vi "testTwoServersSendTelemetryAtSameTime.vi"(8 "error in":errorcluster) -> (0 "error out":errorcluster)   [LabVIEW 2018]
uses:
  <vilib>/addons/_JKI Toolkits/Caraya/classes/Assert/Assert Equal Value_Variant.vi
  src/TcpServer/TcpServer.lvclass
  <vilib>/addons/_JKI Toolkits/Caraya/classes/Test/Test.lvclass
  <vilib>/addons/_JKI Toolkits/Caraya/classes/Assert/Assert.lvclass
panel:
  out "Run Server B error":errorcluster
  out "Run Server A error":errorcluster
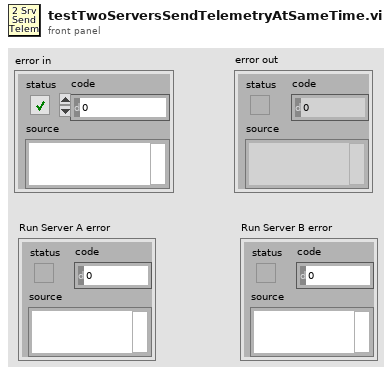
[diagram p1: front panel]
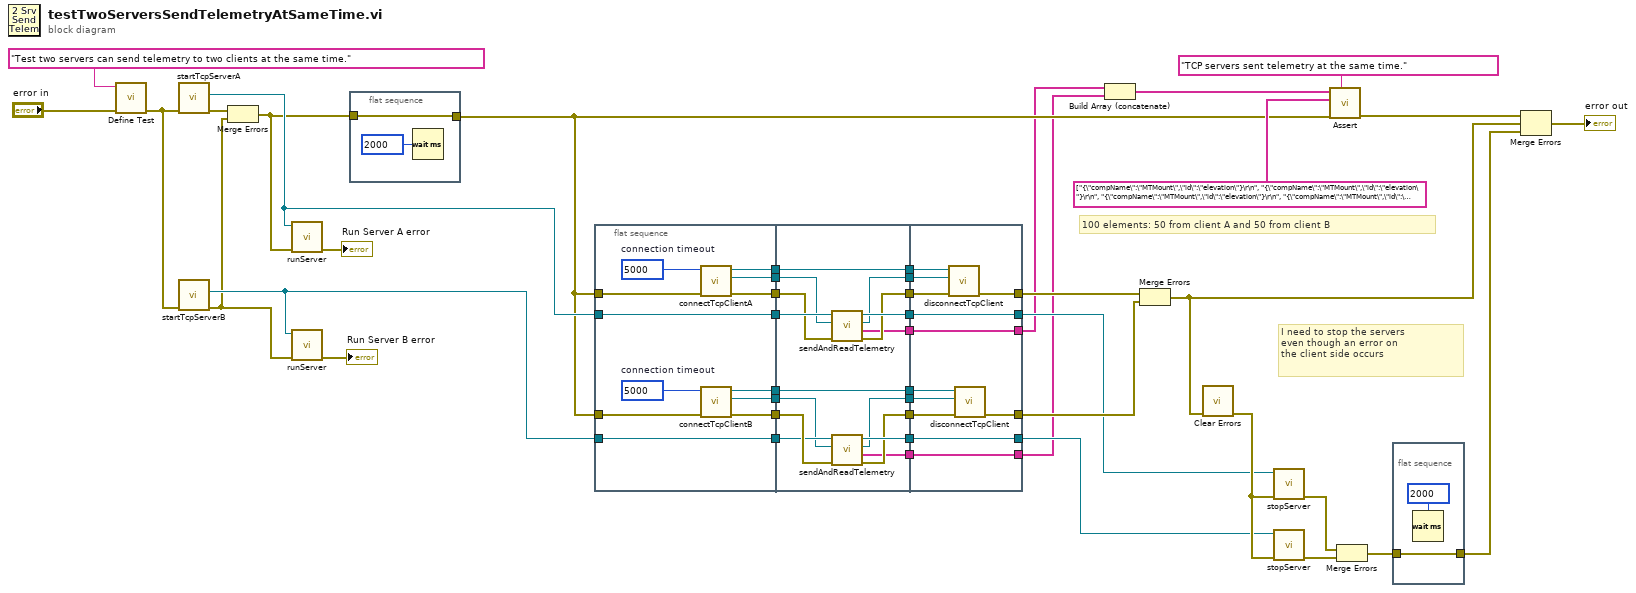
[diagram p0: block diagram]
diagram:
  # "100 elements: 50 from client A and 50 from client B"
  # "I need to stop the servers \neven though an error on \nthe client side occurs"
  n1 = call <vilib>:"Define Test.vi"("error in (no error)"="error in", "Label (VI Title)"="Test two servers can send telemetry to two clients at the same time.") -> ("error out"=w39:errorcluster)  [unwired: 9 in]
  n2 = call "startTcpServerA.vi"("error in (no error)"=w39) -> ("error out"=w35:errorcluster, "TcpServer out"=w34:refnum<class "TcpServer.lvclass">)  [unwired: 8 in, 1 out]
  n3 = call "startTcpServerB.vi"("error in (no error)"=w39) -> ("error out"=w1:errorcluster, "TcpServer out"=w33:refnum<class "TcpServer.lvclass">)  [unwired: 8 in, 1 out]
  n4 = Merge Errors(w35, w1) -> (w2:errorcluster)
  n5 = call "runServer.vi"("error in (no error)"=w2, "TcpServer in"=w34) -> ("error out (no error)"=→"Run Server A error":errorcluster)  [unwired: 8 in, 1 out]
  n6 = call "runServer.vi"("error in (no error)"=w1, "TcpServer in"=w33) -> ("error out (no error)"=→"Run Server B error":errorcluster)  [unwired: 8 in, 1 out]
  n7 = flat-sequence {
    tunnel: [w47] -> w24
    tunnel: w2 -> [w47]
    frame #0 {
      n8 = Wait (ms)(milliseconds to wait=u32 2000) -> ()  [unwired: 1 out]
    }
  }
  n9 = flat-sequence {
    tunnel: w33 -> [w59]
    tunnel: w34 -> [w60]
    tunnel: [w60] -> w29
    tunnel: [w59] -> w28
    tunnel: [w57] -> w27
    tunnel: w24 -> [w58]
    tunnel: [w56] -> w26
    tunnel: [w55] -> w25
    tunnel: w24 -> [w54]
    tunnel: [w53] -> w23
    tunnel: [w52] -> w22
    tunnel: [w51] -> w21
    tunnel: w29 -> [w74]
    tunnel: w28 -> [w69]
    tunnel: w27 -> [w72]
    tunnel: w26 -> [w73]
    tunnel: w25 -> [w76]
    tunnel: w23 -> [w70]
    tunnel: w22 -> [w75]
    tunnel: w21 -> [w67]
    tunnel: [w71] -> w18
    tunnel: [w68] -> w17
    tunnel: [w76] -> w16
    tunnel: [w75] -> w15
    tunnel: [w66] -> w14
    tunnel: [w65] -> w13
    tunnel: [w64] -> w12
    tunnel: [w63] -> w11
    tunnel: [w62] -> w10
    tunnel: [w61] -> w9
    tunnel: w18 -> [w80]
    tunnel: w17 -> [w78]
    tunnel: w16 -> [w86]
    tunnel: w15 -> [w83]
    tunnel: w14 -> [w84]
    tunnel: w13 -> [w81]
    tunnel: w12 -> [w85]
    tunnel: w11 -> [w82]
    tunnel: w10 -> [w79]
    tunnel: w9 -> [w77]
    tunnel: [w88] -> w8
    tunnel: [w87] -> w7
    tunnel: [w80] -> w6
    tunnel: [w79] -> w5
    tunnel: [w78] -> w4
    tunnel: [w77] -> w3
    frame #0 {
      w49 = 5000  # connection timeout
      w50 = 5000  # connection timeout
      n10 = call "connectTcpClientA.vi"("error in (no error)"=w58, "connection timeout (ms)"=w50) -> ("error out"=w57:errorcluster, "tel connection ID A out"=w56:refnum<k5>, "cmd connection ID A out"=w55:refnum<k5>)  [unwired: 7 in]
      n11 = call "connectTcpClientB.vi"("error in (no error)"=w54, "connection timeout (ms)"=w49) -> ("error out"=w53:errorcluster, "tel connection ID B out"=w51:refnum<k5>, "cmd connection ID B out"=w52:refnum<k5>)  [unwired: 7 in]
    }
    frame #1 {
      n12 = call "sendAndReadTelemetry.vi"("error in (no error)"=w72, "tel connection in"=w73, "TcpServer out"=w74) -> ("error out"=w66:errorcluster, "telemetry received"=w62:string[], "tel connection out"=w64:refnum<k5>, "tcpServer out"=w71:refnum<class "TcpServer.lvclass">)  [unwired: 5 in]
      n13 = call "sendAndReadTelemetry.vi"("error in (no error)"=w70, "tel connection in"=w67, "TcpServer out"=w69) -> ("error out"=w65:errorcluster, "telemetry received"=w61:string[], "tel connection out"=w63:refnum<k5>, "tcpServer out"=w68:refnum<class "TcpServer.lvclass">)  [unwired: 5 in]
    }
    frame #2 {
      n14 = call "disconnectTcpClient.vi"("error in (no error)"=w84, "tel connection ID in"=w85, "cmd connection ID in"=w86) -> ("error out"=w88:errorcluster)  [unwired: 8 in]
      n15 = call "disconnectTcpClient.vi"("error in (no error)"=w81, "tel connection ID in"=w82, "cmd connection ID in"=w83) -> ("error out"=w87:errorcluster)  [unwired: 8 in]
    }
  }
  n16 = Build Array (concatenate)(w5, w3) -> (w31:string[])
  n17 = Merge Errors(w8, w7) -> (w37:errorcluster)
  n18 = call <vilib>:"Clear Errors.vi"("error in (no error)"=w37) -> ("error out"=w36:errorcluster)  [unwired: 5 in, 1 out]
  n19 = call "stopServer.vi"("error in (no error)"=w36, "tcpServer in"=w6) -> ("error out"=w44:errorcluster)  [unwired: 8 in, 1 out]
  n20 = call "stopServer.vi"("error in (no error)"=w36, "tcpServer in"=w4) -> ("error out"=w43:errorcluster)  [unwired: 8 in, 1 out]
  n21 = call-poly <vilib>:"Assert.vi"("Label"="TCP servers sent telemetry at the same time.", "error in (no error)"=w24, "Y"=string[] ["{\"compName\":\"MTMount\",\"id\":\"elevation\"}\r\n", "{\"compName\":\"MTMount\",\"id\":\"elevation\"}\r\n", "{\"compName\":\"MTMount\",\"id\":\"elevation\"}\r\n", "{\"compName\":\"MTMount\",\"id\":\"elevation\"}\r\n", "{\"compName\":\"MTMount\",\"id\":\"elevation\"}\r\n", "{\"compName\":\"MTMount\",\"id\":\"elevation\"}\r\n", "{\"compName\":\"MTMount\",\"id\":\"elevation\"}\r\n", "{\"compName\":\"MTMount\",\"id\":\"elevation\"}\r\n", "{\"compName\":\"MTMount\",\"id\":\"elevation\"}\r\n", "{\"compName\":\"MTMount\",\"id\":\"elevation\"}\r\n", "{\"compName\":\"MTMount\",\"id\":\"elevation\"}\r\n", "{\"compName\":\"MTMount\",\"id\":\"elevation\"}\r\n", "{\"compName\":\"MTMount\",\"id\":\"elevation\"}\r\n", "{\"compName\":\"MTMount\",\"id\":\"elevation\"}\r\n", "{\"compName\":\"MTMount\",\"id\":\"elevation\"}\r\n", "{\"compName\":\"MTMount\",\"id\":\"elevation\"}\r\n", "{\"compName\":\"MTMount\",\"id\":\"elevation\"}\r\n", "{\"compName\":\"MTMount\",\"id\":\"elevation\"}\r\n", "{\"compName\":\"MTMount\",\"id\":\"elevation\"}\r\n", "{\"compName\":\"MTMount\",\"id\":\"elevation\"}\r\n", "{\"compName\":\"MTMount\",\"id\":\"elevation\"}\r\n", "{\"compName\":\"MTMount\",\"id\":\"elevation\"}\r\n", "{\"compName\":\"MTMount\",\"id\":\"elevation\"}\r\n", "{\"compName\":\"MTMount\",\"id\":\"elevation\"}\r\n", "{\"compName\":\"MTMount\",\"id\":\"elevation\"}\r\n", "{\"compName\":\"MTMount\",\"id\":\"elevation\"}\r\n", "{\"compName\":\"MTMount\",\"id\":\"elevation\"}\r\n", "{\"compName\":\"MTMount\",\"id\":\"elevation\"}\r\n", "{\"compName\":\"MTMount\",\"id\":\"elevation\"}\r\n", "{\"compName\":\"MTMount\",\"id\":\"elevation\"}\r\n", "{\"compName\":\"MTMount\",\"id\":\"elevation\"}\r\n", "{\"compName\":\"MTMount\",\"id\":\"elevation\"}\r\n", "{\"compName\":\"MTMount\",\"id\":\"elevation\"}\r\n", "{\"compName\":\"MTMount\",\"id\":\"elevation\"}\r\n", "{\"compName\":\"MTMount\",\"id\":\"elevation\"}\r\n", "{\"compName\":\"MTMount\",\"id\":\"elevation\"}\r\n", "{\"compName\":\"MTMount\",\"id\":\"elevation\"}\r\n", "{\"compName\":\"MTMount\",\"id\":\"elevation\"}\r\n", "{\"compName\":\"MTMount\",\"id\":\"elevation\"}\r\n", "{\"compName\":\"MTMount\",\"id\":\"elevation\"}\r\n", "{\"compName\":\"MTMount\",\"id\":\"elevation\"}\r\n", "{\"compName\":\"MTMount\",\"id\":\"elevation\"}\r\n", "{\"compName\":\"MTMount\",\"id\":\"elevation\"}\r\n", "{\"compName\":\"MTMount\",\"id\":\"elevation\"}\r\n", "{\"compName\":\"MTMount\",\"id\":\"elevation\"}\r\n", "{\"compName\":\"MTMount\",\"id\":\"elevation\"}\r\n", "{\"compName\":\"MTMount\",\"id\":\"elevation\"}\r\n", "{\"compName\":\"MTMount\",\"id\":\"elevation\"}\r\n", "{\"compName\":\"MTMount\",\"id\":\"elevation\"}\r\n", "{\"compName\":\"MTMount\",\"id\":\"elevation\"}\r\n", "{\"compName\":\"MTMount\",\"id\":\"elevation\"}\r\n", "{\"compName\":\"MTMount\",\"id\":\"elevation\"}\r\n", "{\"compName\":\"MTMount\",\"id\":\"elevation\"}\r\n", "{\"compName\":\"MTMount\",\"id\":\"elevation\"}\r\n", "{\"compName\":\"MTMount\",\"id\":\"elevation\"}\r\n", "{\"compName\":\"MTMount\",\"id\":\"elevation\"}\r\n", "{\"compName\":\"MTMount\",\"id\":\"elevation\"}\r\n", "{\"compName\":\"MTMount\",\"id\":\"elevation\"}\r\n", "{\"compName\":\"MTMount\",\"id\":\"elevation\"}\r\n", "{\"compName\":\"MTMount\",\"id\":\"elevation\"}\r\n", "{\"compName\":\"MTMount\",\"id\":\"elevation\"}\r\n", "{\"compName\":\"MTMount\",\"id\":\"elevation\"}\r\n", "{\"compName\":\"MTMount\",\"id\":\"elevation\"}\r\n", "{\"compName\":\"MTMount\",\"id\":\"elevation\"}\r\n", "{\"compName\":\"MTMount\",\"id\":\"elevation\"}\r\n", "{\"compName\":\"MTMount\",\"id\":\"elevation\"}\r\n", "{\"compName\":\"MTMount\",\"id\":\"elevation\"}\r\n", "{\"compName\":\"MTMount\",\"id\":\"elevation\"}\r\n", "{\"compName\":\"MTMount\",\"id\":\"elevation\"}\r\n", "{\"compName\":\"MTMount\",\"id\":\"elevation\"}\r\n", "{\"compName\":\"MTMount\",\"id\":\"elevation\"}\r\n", "{\"compName\":\"MTMount\",\"id\":\"elevation\"}\r\n", "{\"compName\":\"MTMount\",\"id\":\"elevation\"}\r\n", "{\"compName\":\"MTMount\",\"id\":\"elevation\"}\r\n", "{\"compName\":\"MTMount\",\"id\":\"elevation\"}\r\n", "{\"compName\":\"MTMount\",\"id\":\"elevation\"}\r\n", "{\"compName\":\"MTMount\",\"id\":\"elevation\"}\r\n", "{\"compName\":\"MTMount\",\"id\":\"elevation\"}\r\n", "{\"compName\":\"MTMount\",\"id\":\"elevation\"}\r\n", "{\"compName\":\"MTMount\",\"id\":\"elevation\"}\r\n", "{\"compName\":\"MTMount\",\"id\":\"elevation\"}\r\n", "{\"compName\":\"MTMount\",\"id\":\"elevation\"}\r\n", "{\"compName\":\"MTMount\",\"id\":\"elevation\"}\r\n", "{\"compName\":\"MTMount\",\"id\":\"elevation\"}\r\n", "{\"compName\":\"MTMount\",\"id\":\"elevation\"}\r\n", "{\"compName\":\"MTMount\",\"id\":\"elevation\"}\r\n", "{\"compName\":\"MTMount\",\"id\":\"elevation\"}\r\n", "{\"compName\":\"MTMount\",\"id\":\"elevation\"}\r\n", "{\"compName\":\"MTMount\",\"id\":\"elevation\"}\r\n", "{\"compName\":\"MTMount\",\"id\":\"elevation\"}\r\n", "{\"compName\":\"MTMount\",\"id\":\"elevation\"}\r\n", "{\"compName\":\"MTMount\",\"id\":\"elevation\"}\r\n", "{\"compName\":\"MTMount\",\"id\":\"elevation\"}\r\n", "{\"compName\":\"MTMount\",\"id\":\"elevation\"}\r\n", "{\"compName\":\"MTMount\",\"id\":\"elevation\"}\r\n", "{\"compName\":\"MTMount\",\"id\":\"elevation\"}\r\n", "{\"compName\":\"MTMount\",\"id\":\"elevation\"}\r\n", "{\"compName\":\"MTMount\",\"id\":\"elevation\"}\r\n", "{\"compName\":\"MTMount\",\"id\":\"elevation\"}\r\n", "{\"compName\":\"MTMount\",\"id\":\"elevation\"}\r\n"] ("appended array"), "X"=w31) -> ("error out"=w32:errorcluster)  [unwired: 7 in]
  n22 = Merge Errors(w44, w43) -> (w42:errorcluster)
  n23 = flat-sequence {
    tunnel: w42 -> [w89]
    tunnel: [w89] -> w38
    frame #0 {
      n24 = Wait (ms)(milliseconds to wait=u32 2000) -> ()  [unwired: 1 out]
    }
  }
  n25 = Merge Errors(w32, w37, w38) -> (→"error out":errorcluster)
